vi "create_LS350_Data_header.vi"() -> (3 "String":string)   [LabVIEW 2019]
uses:
  Instrument_Setup.vi
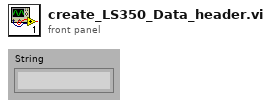
[diagram p1: front panel]
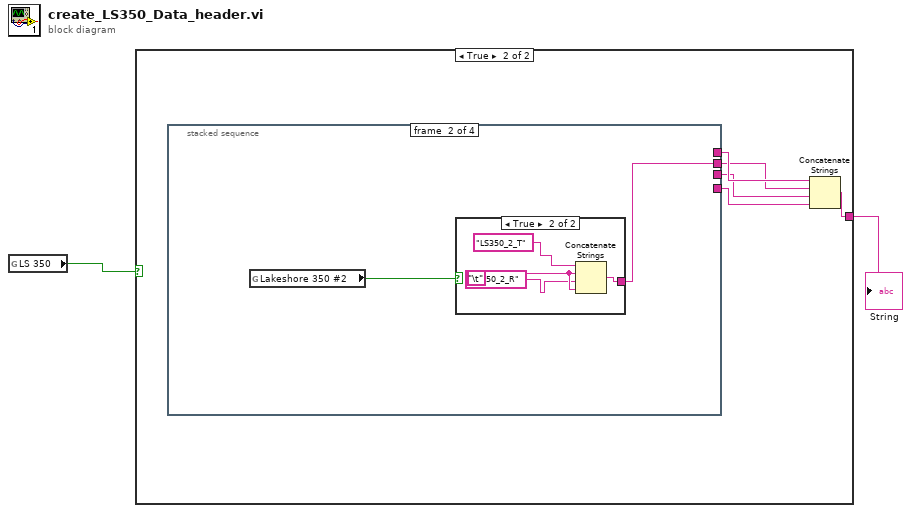
[diagram p0: block diagram]
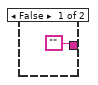
[diagram p2: hidden frame]
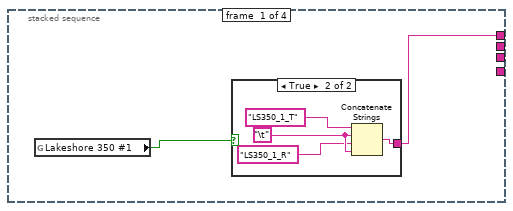
[diagram p3: hidden frame]
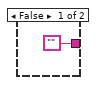
[diagram p4: hidden frame]
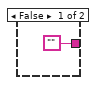
[diagram p5: hidden frame]
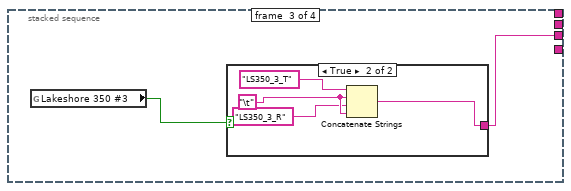
[diagram p6: hidden frame]
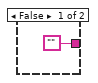
[diagram p7: hidden frame]
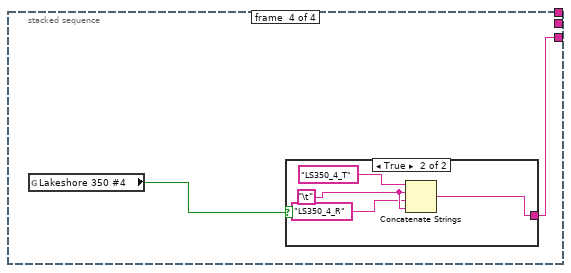
[diagram p8: hidden frame]
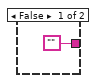
[diagram p9: hidden frame]
diagram:
  n1 = global read "Instrument_Setup.vi" "LS 350"() -> (w1:bool)
  n2 = case shown="True" w1 {
    tunnel: ["" w4] -> w2
    frame False {
    }
    frame True {
      n3 = stacked-sequence {
        tunnel: [w9 _ _ _] -> w8
        tunnel: [_ w16 _ _] -> w7
        tunnel: [_ _ w23 _] -> w6
        tunnel: [_ _ _ w30] -> w5
        frame #0 {
          n4 = global read "Instrument_Setup.vi" "Lakeshore 350 #1"() -> (w10:bool)
          n5 = case shown="True" w10 {
            tunnel: ["" w15] -> w9
            frame False {
            }
            frame True {
              w13 = "\t"
              n6 = Concatenate Strings("LS350_1_T", w13, "LS350_1_R", w13) -> (w15:string)
            }
          }
        }
        frame #1 {
          n7 = global read "Instrument_Setup.vi" "Lakeshore 350 #2"() -> (w17:bool)
          n8 = case shown="True" w17 {
            tunnel: ["" w22] -> w16
            frame False {
            }
            frame True {
              w21 = "\t"
              n9 = Concatenate Strings("LS350_2_T", w21, "LS350_2_R", w21) -> (w22:string)
            }
          }
        }
        frame #2 {
          n10 = global read "Instrument_Setup.vi" "Lakeshore 350 #3"() -> (w24:bool)
          n11 = case shown="True" w24 {
            tunnel: ["" w26] -> w23
            frame False {
            }
            frame True {
              w28 = "\t"
              n12 = Concatenate Strings("LS350_3_T", w28, "LS350_3_R", w28) -> (w26:string)
            }
          }
        }
        frame #3 {
          n13 = global read "Instrument_Setup.vi" "Lakeshore 350 #4"() -> (w31:bool)
          n14 = case shown="True" w31 {
            tunnel: ["" w33] -> w30
            frame False {
            }
            frame True {
              w35 = "\t"
              n15 = Concatenate Strings("LS350_4_T", w35, "LS350_4_R", w35) -> (w33:string)
            }
          }
        }
      }
      n16 = Concatenate Strings(w8, w7, w6, w5) -> (w4:string)
    }
  }
  "String" <- w2
